vi "PH_4_Pos_Selector.Evt Call Relative Mode.vi"(0 "i ref in":refnum<vi>, 1 "4 Pos instance":string, 3 "Relative Mode?":bool, 5 "error in":errorcluster) -> (14 "i ref out":refnum<vi>, 19 "error out":errorcluster)   [LabVIEW 2014, in "PH_4_Pos_Selector.lvlib"]
uses:
  PH_4_Pos_Selector.lvlib
  CSCore/CSSystem/CoreLib/CoreLib.short 2 byte array.vi
  CSCore/CSSystem/CoreLib/CoreLib.lvlib
  CSCore/BaseProcess/BaseProcess.lvlib
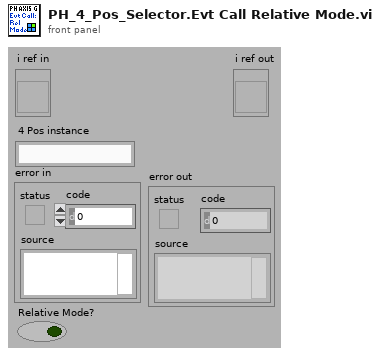
[diagram p1: front panel]
types:
  T1 = typedef "CoreDefs.rawDataType.ctl" = i8[]
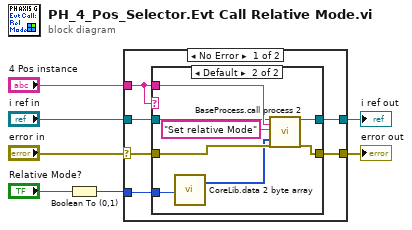
[diagram p0: block diagram]
diagram:
  n1 = Boolean To (0,1)(Boolean="Relative Mode?") -> (0, 1=w1:i16)
  n2 = case shown="No Error" "error in" {
    selector: "error in" -> [w9 w24]
    tunnel: [w13 w24] -> w4
    tunnel: "4 Pos instance" -> [w8 _]
    tunnel: "i ref in" -> [w12 w25]
    tunnel: [w11 w25] -> w6
    tunnel: w1 -> [w10 _]
    frame No Error {
      n3 = case shown="Default" w8 {
        tunnel: [w15 w23] -> w13
        tunnel: w8 -> [_ w21]
        tunnel: w9 -> [w15 w20]
        tunnel: w12 -> [w14 w19]
        tunnel: [w14 w18] -> w11
        tunnel: w10 -> [_ w17]
        frame "N/A" {
        }
        frame Default {
          n4 = call-poly "CoreLib.data 2 byte array.vi"("i16"=w17) -> ("byteArray out"=w16:T1)  [unwired: 18 in]
          n5 = call "BaseProcess.call process 2.vi"("i ref in"=w19, "Object"=w21, "Selector"="Set relative Mode", "Data"=w16, "error in (no error)"=w20) -> ("i ref out"=w18:refnum<vi>, "error out"=w23:errorcluster)  [unwired: 13 in]
        }
      }
    }
    frame Error {
    }
  }
  "i ref out" <- w6
  "error out" <- w4
